vi "Write DAQ FIFO.vi"(6 "FIFO Timestamps":T2, 7 "Channel Index":i32, 8 "error in (no error)":errorcluster, 9 "Timeout (ms)":i32=200, 10 "Data In":T1[](array[typedef]), 11 "CIFCorePlugin in":refnum<class "CIFCorePlugin.lvclass">) -> (0 "error out":errorcluster, 1 "timed out?":bool, 2 "Data Out":T1[](array[typedef]), 3 "CIFCorePlugin out":refnum<class "CIFCorePlugin.lvclass">)   [LabVIEW 2021, in "CIFCorePlugin.lvclass"]
uses:
  CIFCorePlugin.lvclass
  CIFCorePlugin.lvclass/CIFCorePlugin.ctl
  Channels/CIFChannelMng/CIFChannelMng.lvclass
  Channels/CIFChannels/CIFChannels.lvclass
  Channels/ChannelCommon/typedef/TimeStamps.ctl
  Channels/ChannelCommon/ChannelCommon.lvlib
  Channels/ChannelCommon/typedef/Datatype Waveform.ctl
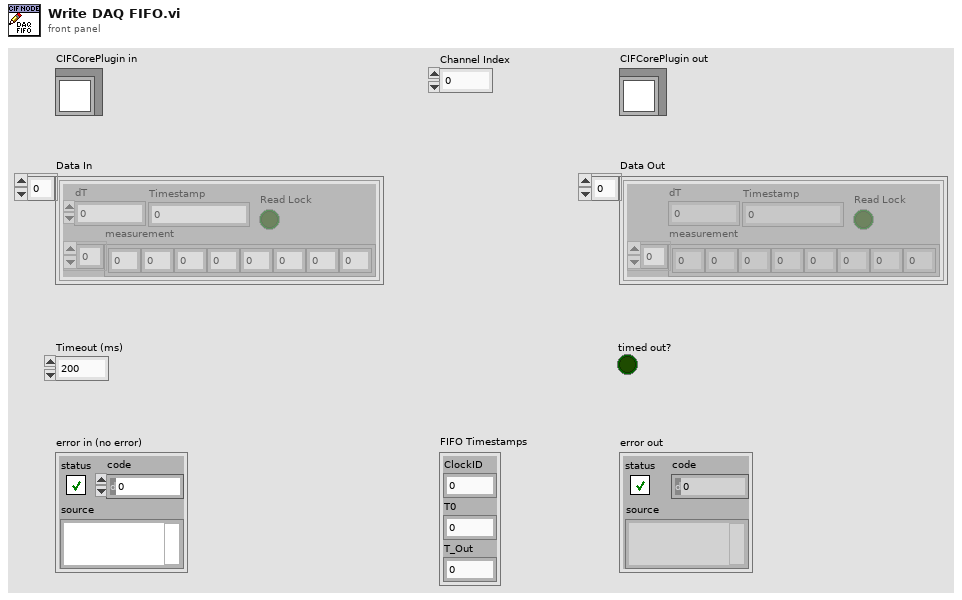
[diagram p1: front panel]
types:
  T1 = typedef "ChannelCommon.lvlib/Datatype Waveform.ctl" = cluster{"measurement":dbl[], "dT":dbl, "Timestamp":u64, "Read Lock":bool}
  T2 = typedef "ChannelCommon.lvlib/TimeStamps.ctl" = cluster{"ClockID":u8, "T0":u64, "T_Out":u64}
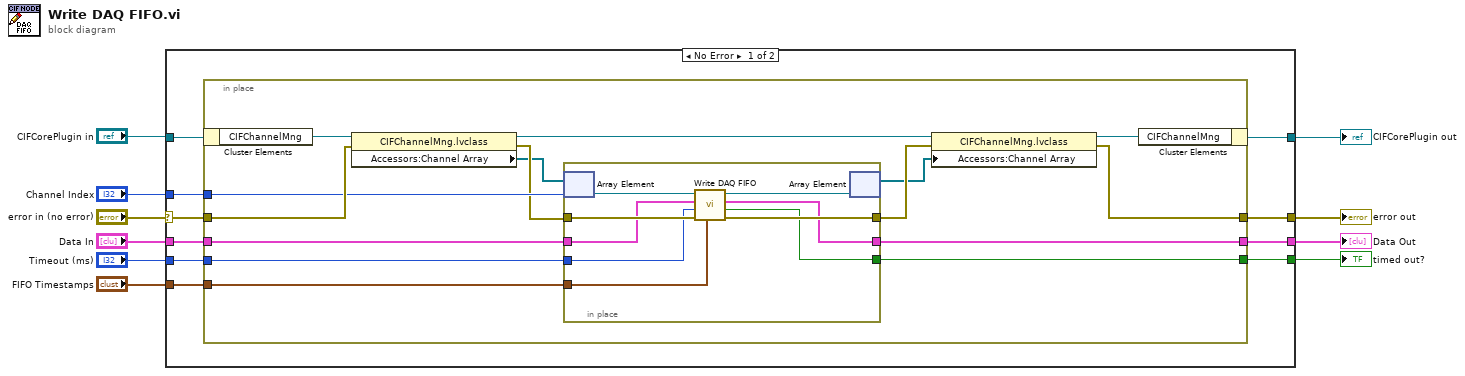
[diagram p0: block diagram]
diagram:
  n1 = case shown="No Error" "error in (no error)" {
    selector: "error in (no error)" -> [w20 w47]
    tunnel: [w19 w47] -> w8
    tunnel: [w17 w46] -> w9
    tunnel: "CIFCorePlugin in" -> [w18 w46]
    tunnel: "Channel Index" -> [w16 _]
    tunnel: "Data In" -> [w15 w45]
    tunnel: "Timeout (ms)" -> [w14 _]
    tunnel: [w13 _] -> w4
    tunnel: "FIFO Timestamps" -> [w12 _]
    tunnel: [w11 w45] -> w1
    frame No Error {
      n2 = in-place {
        in-place-border: w20 -> [w33]
        in-place-border: [w26] -> w19
        in-place-border: w16 -> [w32]
        in-place-border: w15 -> [w25]
        in-place-border: w14 -> [w24]
        in-place-border: [w23] -> w13
        in-place-border: w12 -> [w22]
        in-place-border: [w21] -> w11
        n3 = in-place-cluster #1(w18) -> ("CIFChannelMng"=w35:refnum<class "CIFChannelMng.lvclass">)
        n4 = property class="CIFChannelMng.lvclass"(reference=w35, error in=w33) -> (reference out=w31:refnum<class "CIFChannelMng.lvclass">, error out=w30:errorcluster, "Accessors:Channel Array"=w28:refnum<class "CIFChannels.lvclass">[])
        n5 = in-place {
          in-place-border: w30 -> [w43]
          in-place-border: [w42] -> w29
          in-place-border: w25 -> [w40]
          in-place-border: w24 -> [w39]
          in-place-border: [w38] -> w23
          in-place-border: w22 -> [w37]
          in-place-border: [w36] -> w21
          n6 = in-place-array #2(w28, w32) -> (w44:refnum<class "CIFChannels.lvclass">)
          n7 = call-dynamic "Write DAQ FIFO.vi"("FIFO Timestamps"=w37, "error in (no error)"=w43, "Timeout (ms)"=w39, "Data In"=w40, "CIFChannels in"=w44) -> ("error out"=w42:errorcluster, "timed out?"=w38:bool, "Data Out"=w36:T1[], "CIFChannels out"=w41:refnum<class "CIFChannels.lvclass">)  [unwired: 3 in]
          n8 = in-place-array #2(w41) -> (w27:refnum<class "CIFChannels.lvclass">[])  [unwired: 1 out]
        }
        n9 = property class="CIFChannelMng.lvclass"(reference=w31, error in=w29, "Accessors:Channel Array"=w27) -> (reference out=w34:refnum<class "CIFChannelMng.lvclass">, error out=w26:errorcluster)
        n10 = in-place-cluster #1("CIFChannelMng"=w34) -> (w17:refnum<class "CIFCorePlugin.lvclass">)
      }
    }
    frame Error {
    }
  }
  "error out" <- w8
  "CIFCorePlugin out" <- w9
  "timed out?" <- w4
  "Data Out" <- w1
